vi "05TRM500_V2.vi"() -> ()   [LabVIEW 2020]
uses:
  <vilib>/Utility/error.llb/DialogType.ctl
  <vilib>/DAQmx/read.llb/DAQmx Read (Digital 1D U8 1Chan NSamp).vi
  <vilib>/Instr/_visa.llb/VISA Configure Serial Port (Serial Instr).vi
  <vilib>/DAQmx/create/channels.llb/DAQmx Create Channel (DI-Digital Input).vi
  <vilib>/DAQmx/configure/timing.llb/DAQmx Timing (Change Detection).vi
  <vilib>/DAQmx/miscellaneous.llb/DAQmx Fill In Error Info.vi
  <vilib>/ErrorRing/Error Ring.xnode
panel:
  in  "lines":tag="cDAQ1Mod1/port0/line0"
  in  "Tab Control":T1(tab)
  in  "INC DOWN":bool
  in  "INC UP":bool
  in  "MPH DOWN":bool
  in  "MPH UP":bool
  out "INC":dbl min=0.0 max=12.0 step=0.1 format="%.1g"
  out "MPH":dbl min=0.0 max=12.0 step=0.1 format="%.1g"
  out "Reply":string
  out "Error":string
  out "Directory":path
  out "Stopping":bool
  in  "Command":string
  in  "Insert Command":bool
  in  "Wait":bool
  out "Part":string
  in  "STOP":bool
  in  "Port":refnum<visa-resource-name>="COM8"
  in  "milliseconds to wait":u32
  out "Data":T2
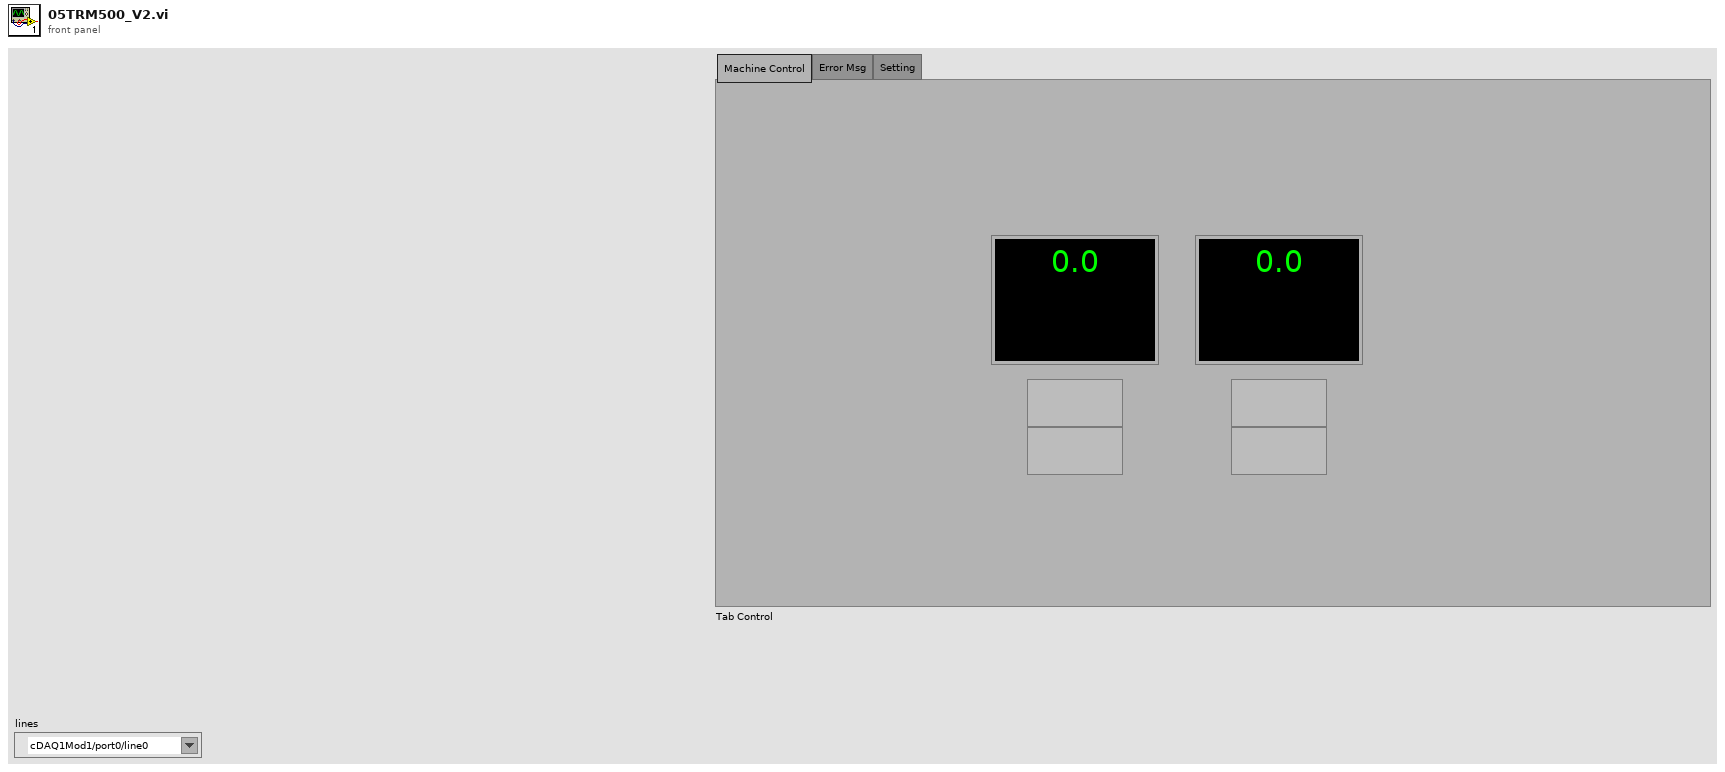
[diagram p1: front panel]
types:
  T1 = enum32{"Machine Control", "Error Msg", "Setting"}
  T2 = cluster{"err":i32[], "vin":i32, "vbus":i32, "amps":i32, "iamp":i32, "mph":i32, "inc":i32}
  T3 = enum16{"Initialize", "Next", "Send RSET", "Set MPH", "Set INC", "Part to 0"}
  T4 = enum16{"err", "mph:", "inc:", "cnfg:", "loop:", "type", "ver", "part:", "led2:", "xmph", "led1", "ptmp", "mtmp", "vbus", "iamp", "vin", "amps", "RSET", "ramp:", "res:", "rng:", "rpm"}[]
  T5 = typedef "DialogType.ctl" = u16
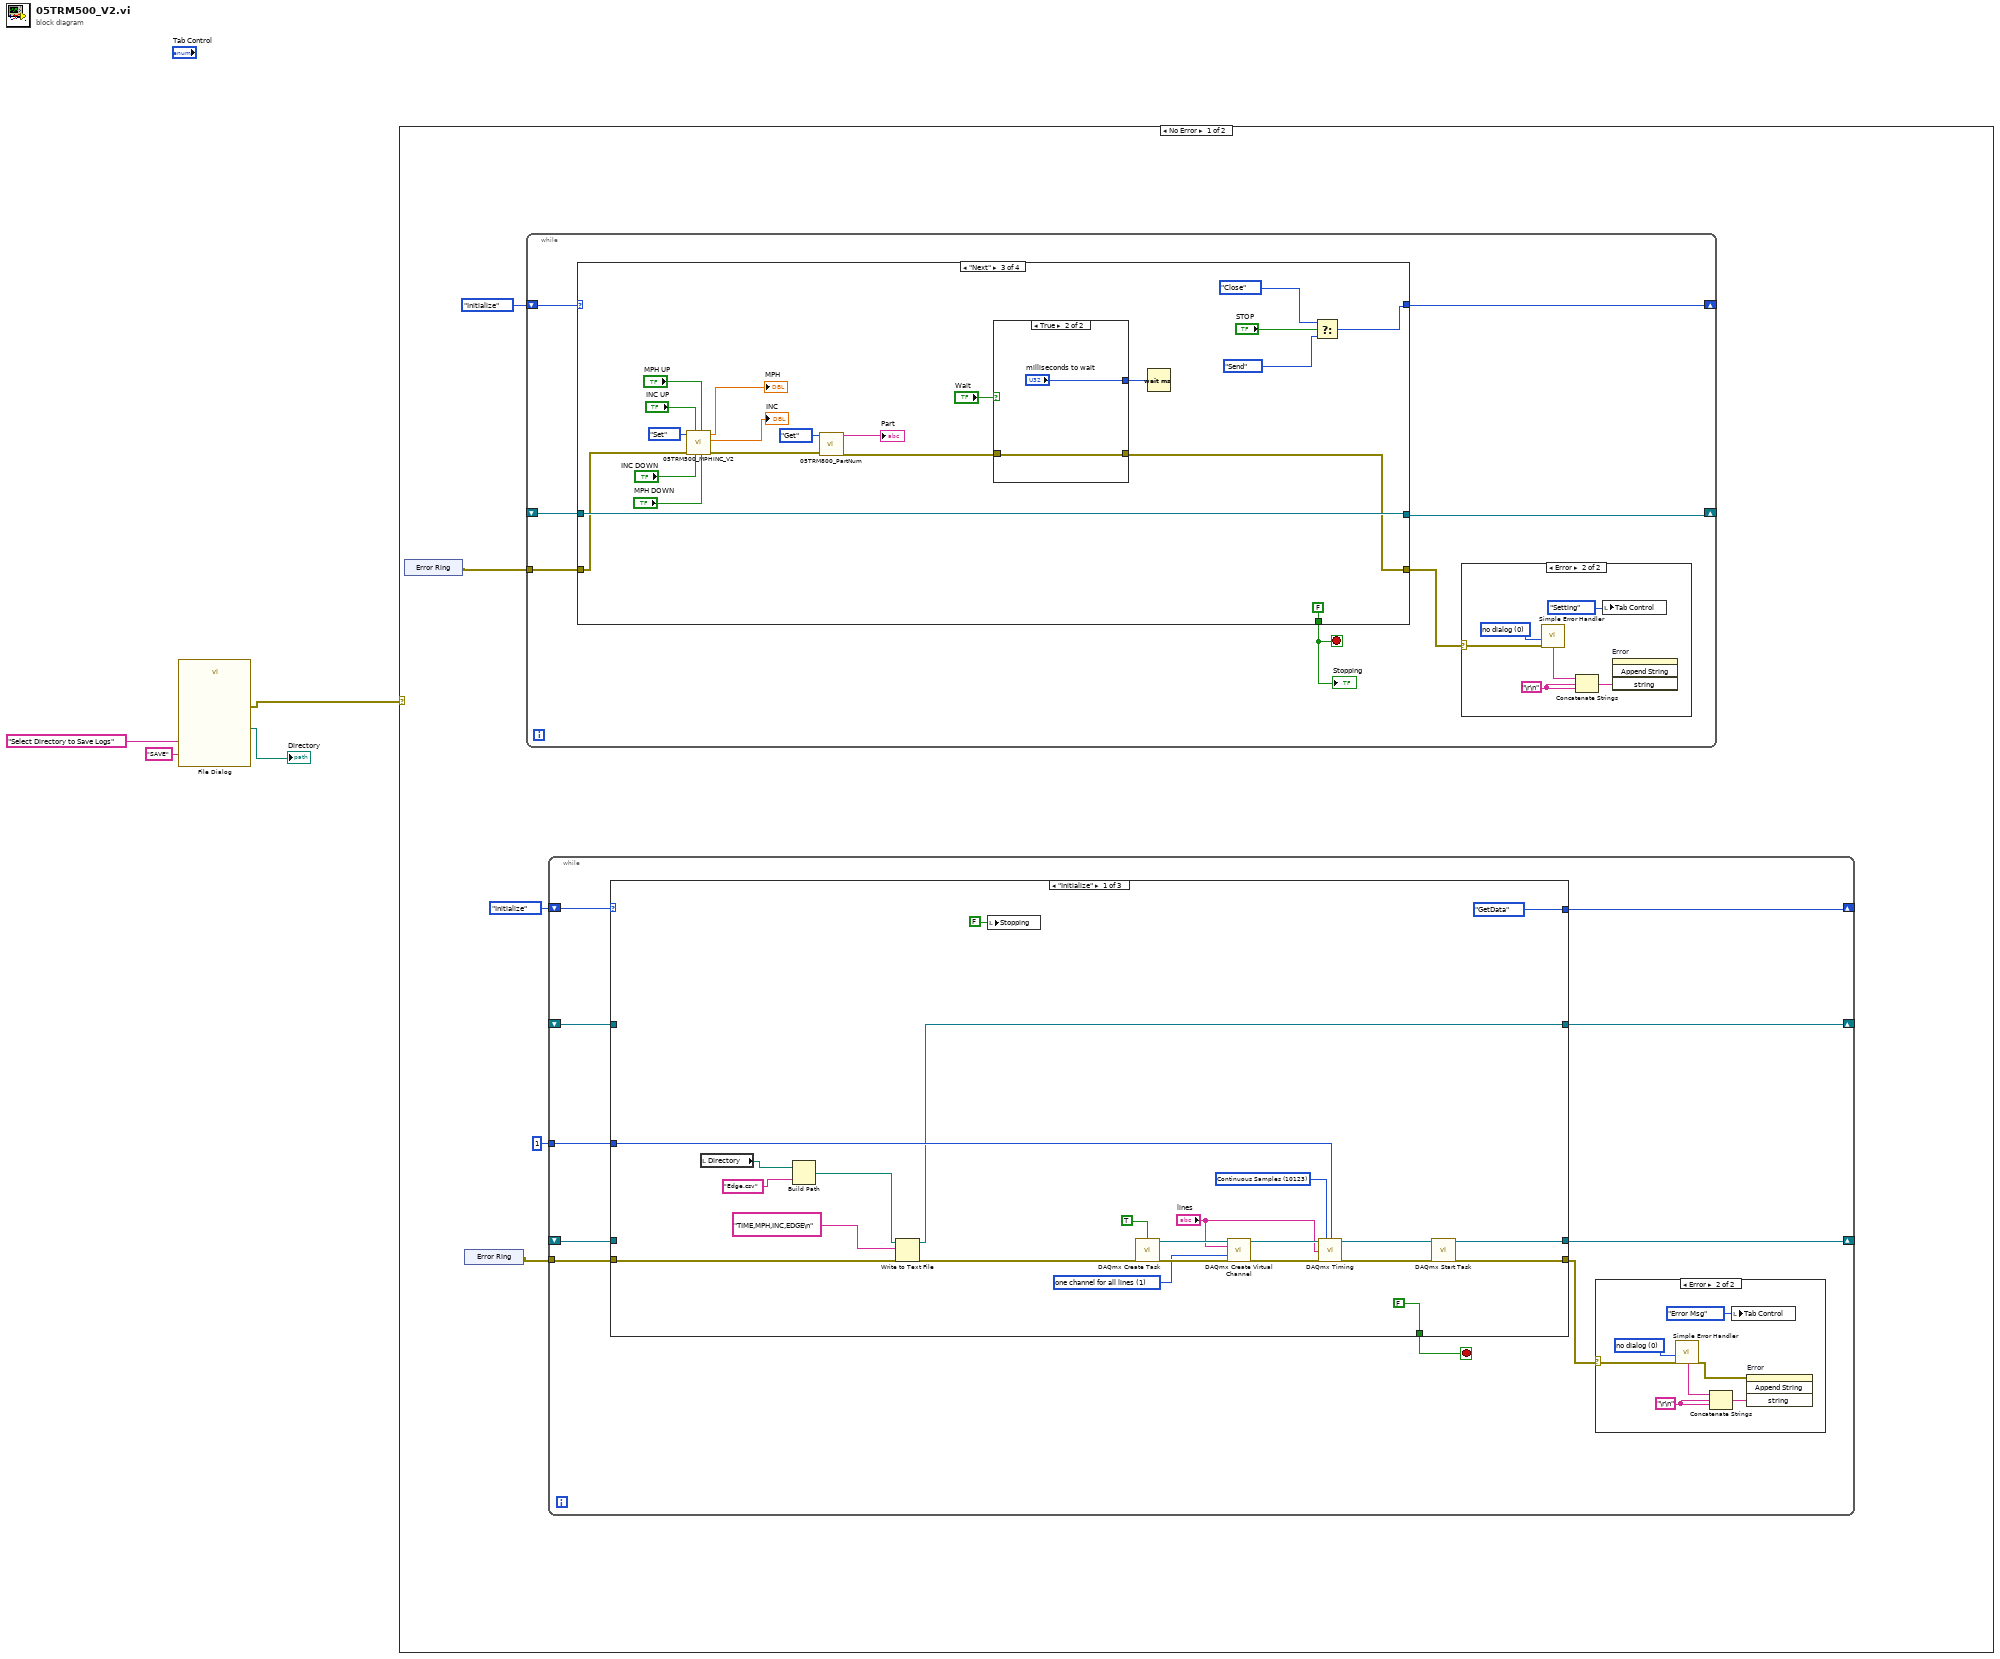
[diagram p0: block diagram]
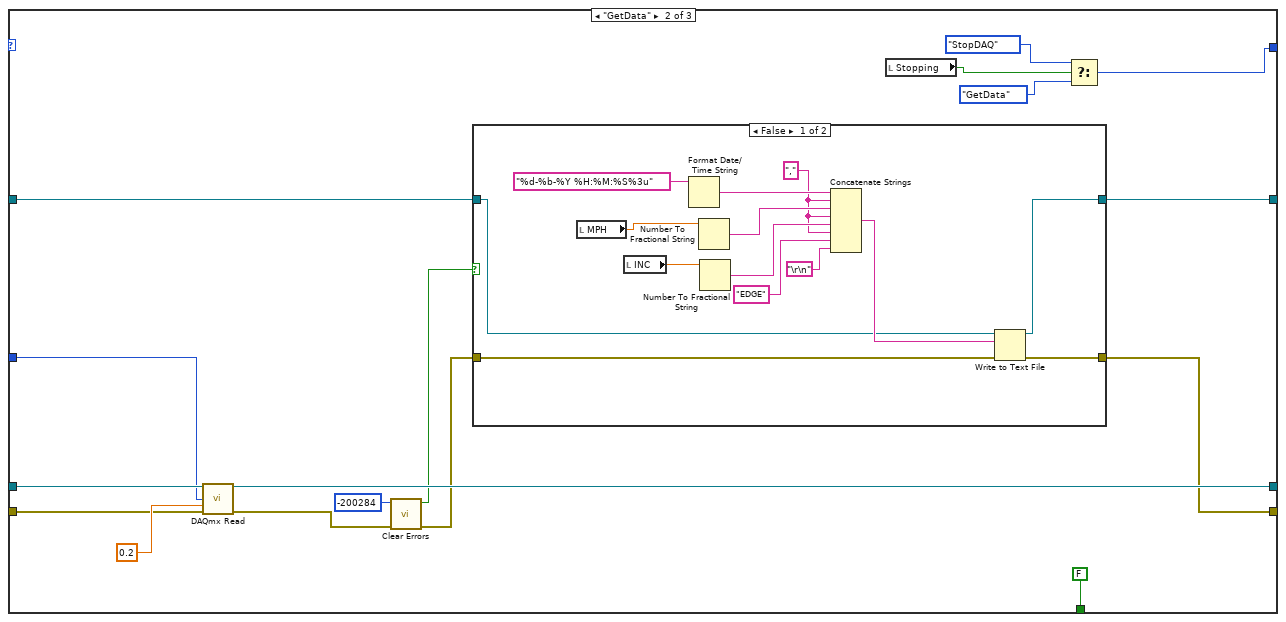
[diagram p3: hidden frame]
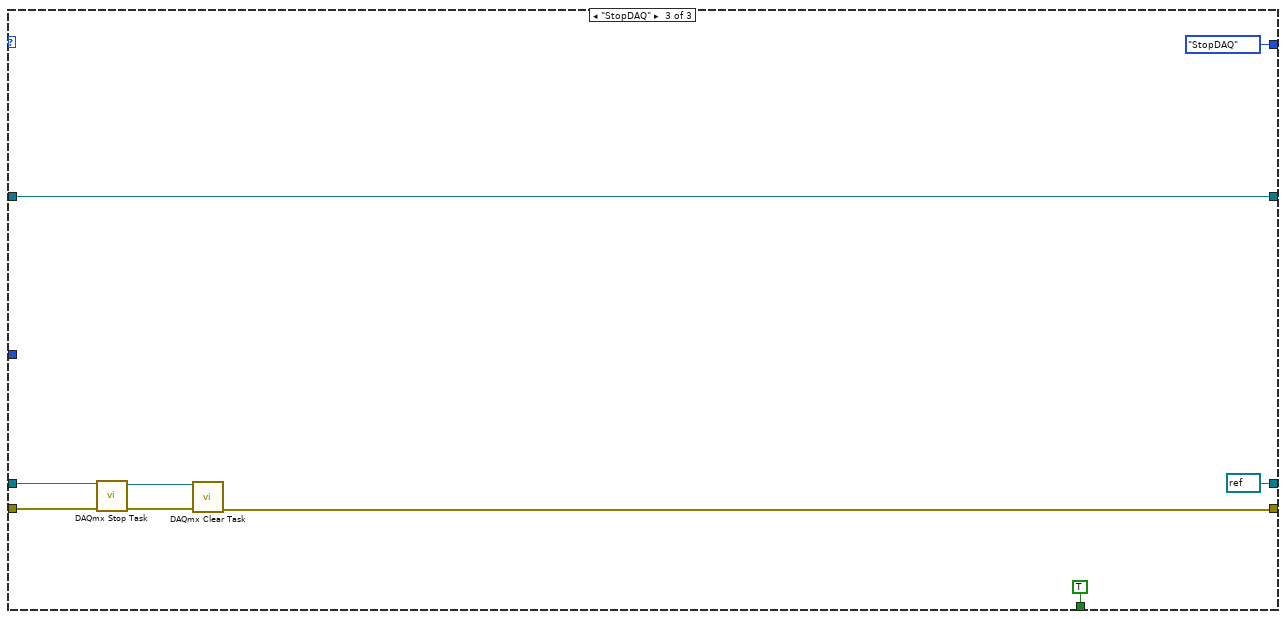
[diagram p5: hidden frame]
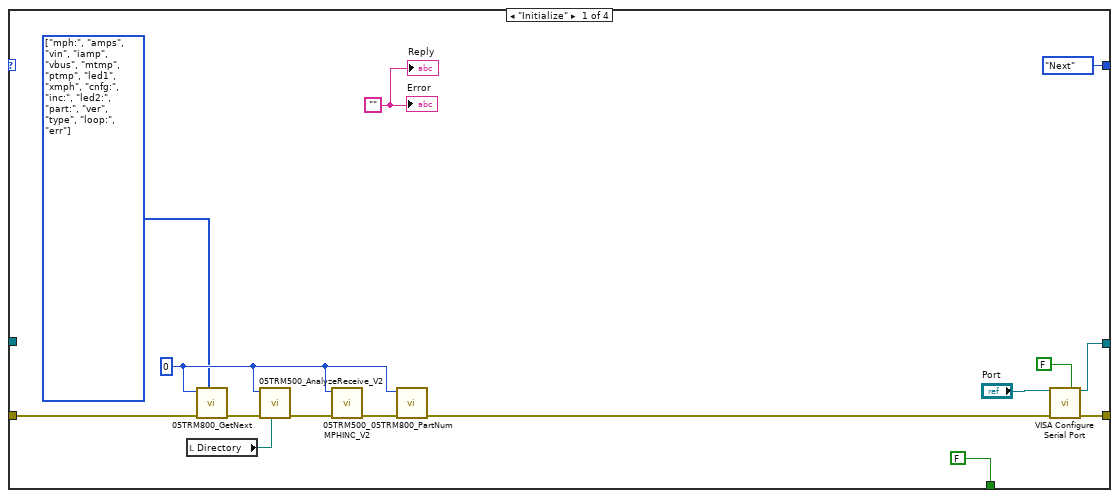
[diagram p7: hidden frame]
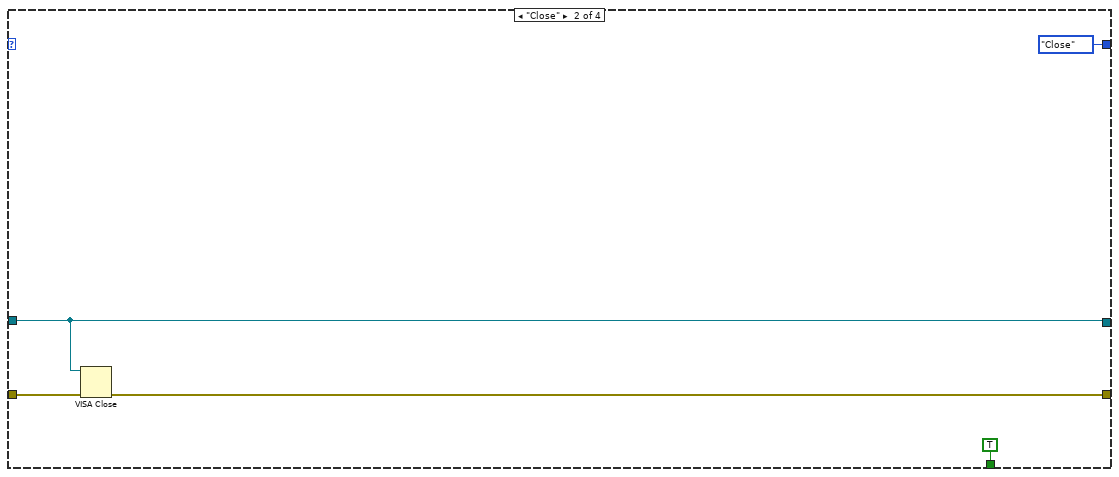
[diagram p8: hidden frame]
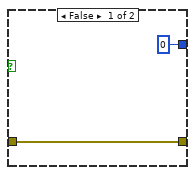
[diagram p9: hidden frame]
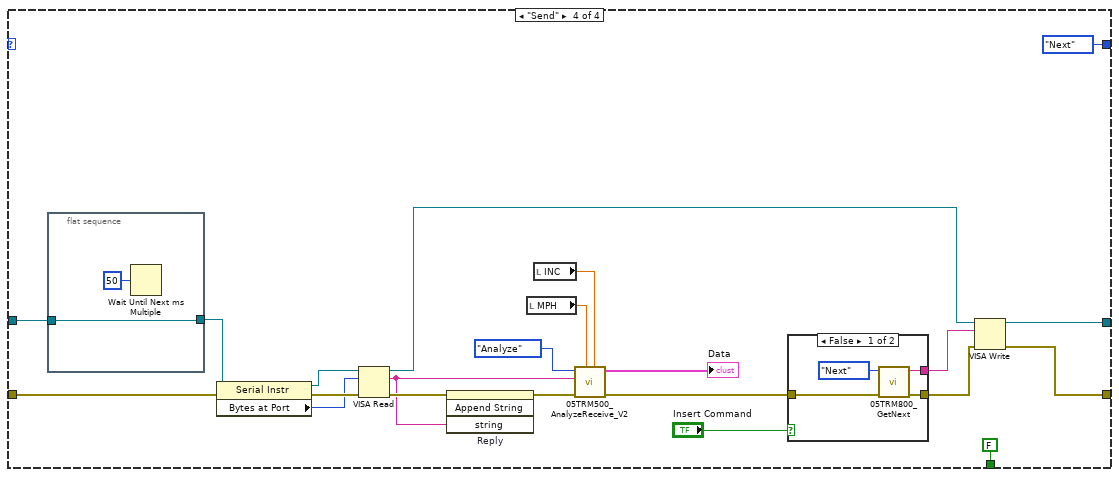
[diagram p10: hidden frame]
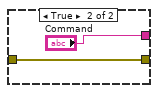
[diagram p11: hidden frame]
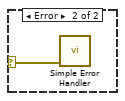
[diagram p12: hidden frame]
diagram:
  n1 = call "File Dialog"("prompt"="Select Directory to Save Logs", "button label"="SAVE") -> ("selected path"=→"Directory":path, "error out"=w4:errorcluster)  [unwired: 10 in, 2 out]
  n2 = case shown="No Error" w4 {
    selector: w4 -> [_ w182]
    frame No Error {
      n3 = xnode "Error Ring"() -> ("error out"=w6:errorcluster)
      n4 = xnode "Error Ring"() -> ("error out"=w5:errorcluster)
      n5 = while {
        shift-right: [w99] -> _
        shift-left: enum16{"Initialize", "Close", "Next", "Send"}."Initialize" -> [w100]
        tunnel: w6 -> [w98]
        shift-right: [w96] -> _
        shift-left: _ -> [w95]
        stop <- w94 stop-if-true
        n6 = case shown="\"Next\"" w100 {
          tunnel: [enum16{"Initialize", "Close", "Next", "Send"}."Next" enum16{"Initialize", "Close", "Next", "Send"}."Close" w145 enum16{"Initialize", "Close", "Next", "Send"}."Next"] -> w99
          tunnel: [FALSE TRUE FALSE FALSE] -> w94
          tunnel: w98 -> [w115 w125 w140 w171]
          tunnel: [w120 w123 w129 w164] -> w97
          tunnel: [w117 w124 w144 w165] -> w96
          tunnel: w95 -> [_ w124 w144 w173]
          frame "Initialize" {
            w109 = T4 [enum."mph:", enum."amps", enum."vin", enum."iamp", enum."vbus", enum."mtmp", enum."ptmp", enum."led1", enum."xmph", enum."cnfg:", enum."inc:", enum."led2:", enum."part:", enum."ver", enum."type", enum."loop:", enum."err"] items=["err", "mph:", "inc:", "cnfg:", "loop:", "type", "ver", "part:", "led2:", "xmph", "led1", "ptmp", "mtmp", "vbus", "iamp", "vin", "amps", "RSET", "ramp:", "res:", "rng:", "rpm"] ("Pattern")
            w112 = u16 0
            w116 = ""
            n7 = local read "Directory"() -> (w107:path)
            n8 = call "05TRM800_GetNext.vi"("Pattern"=w109, "error in (no error)"=w115, "Enum"=w112) -> ("error out"=w114:errorcluster)  [unwired: 7 in, 1 out]
            n9 = call "05TRM500_AnalyzeReceive_V2.vi"("Directory"=w107, "error in (no error)"=w114, "Enum"=w112) -> ("error out"=w113:errorcluster)  [unwired: 7 in, 1 out]
            n10 = call "05TRM500_MPHINC_V2.vi"("error in (no error)"=w113, "Enum"=w112) -> ("error out"=w111:errorcluster)  [unwired: 7 in, 2 out]
            n11 = call "05TRM800_PartNum.vi"("error in (no error)"=w111, "Enum"=w112) -> ("error out"=w110:errorcluster)  [unwired: 8 in, 1 out]
            n12 = call-poly "VISA Configure Serial Port"("VISA resource name"="Port", "Enable Termination\nChar (T)"=FALSE ("Enable Termination\nChar (T)"), "error in (no error)"=w110) -> ("VISA resource name out"=w117:refnum<visa-resource-name>, "error out"=w120:errorcluster)  [unwired: 11 in]
            "Error" <- w116
            "Reply" <- w116
          }
          frame "Close" {
            n13 = VISA Close(VISA resource name=w124, error in (no error)=w125) -> (error out=w123:errorcluster)
          }
          frame "Next" {
            n14 = call "05TRM500_MPHINC_V2.vi"("MPH DOWN"="MPH DOWN", "MPH UP"="MPH UP", "INC DOWN"="INC DOWN", "INC UP"="INC UP", "error in (no error)"=w140, "Enum"=enum16{"Initialize", "Set"}."Set") -> ("error out"=w133:errorcluster, "INC"=→"INC":dbl, "MPH"=→"MPH":dbl)  [unwired: 3 in]
            n15 = call "05TRM800_PartNum.vi"("error in (no error)"=w133, "Enum"=enum16{"Initialize", "Get", "Input"}."Get") -> ("error out"=w130:errorcluster, "Part Num"=→"Part":string)  [unwired: 8 in]
            n16 = case shown="True" "Wait" {
              tunnel: w130 -> [w149 w151]
              tunnel: [w149 w151] -> w129
              tunnel: [u32 0 ("milliseconds to wait") "milliseconds to wait"] -> w128
              frame False {
              }
              frame True {
              }
            }
            n17 = Wait (ms)(milliseconds to wait=w128) -> ()  [unwired: 1 out]
            n18 = Select(t=enum16{"Initialize", "Close", "Next", "Send"}."Close", s="STOP", f=enum16{"Initialize", "Close", "Next", "Send"}."Send") -> (s? t:f=w145:enum16{"Initialize", "Close", "Next", "Send"})
          }
          frame "Send" {
            n19 = flat-sequence {
              tunnel: w173 -> [w180]
              tunnel: [w180] -> w172
              frame #0 {
                n20 = Wait Until Next ms Multiple(millisecond multiple=u32 50) -> ()  [unwired: 1 out]
              }
            }
            n21 = property class="Serial Instr"(reference=w172, error in=w171) -> (reference out=w169:refnum<visa-resource-name>, error out=w170:errorcluster, "Bytes at Port"=w168:u32)
            n22 = VISA Read(VISA resource name=w169, byte count=w168, error in (no error)=w170) -> (VISA resource name out=w166:refnum<visa-resource-name>, read buffer=w157:string, error out=w167:errorcluster)  [unwired: 1 out]
            n23 = invoke on="Reply" class="Str" method="Append String"(error in=w167, "string"=w157) -> (error out=w159:errorcluster)  [unwired: 2 in, 3 out]
            n24 = local read "MPH"() -> (w153:dbl)
            n25 = local read "INC"() -> (w152:dbl)
            n26 = call "05TRM500_AnalyzeReceive_V2.vi"("INC"=w152, "MPH"=w153, "error in (no error)"=w159, "String"=w157, "Enum"=enum16{"Initialize", "Analyze"}."Analyze") -> ("error out"=w158:errorcluster, "Data"=→"Data":T2)  [unwired: 5 in]
            n27 = case shown="False" "Insert Command" {
              tunnel: [w177 "Command"] -> w161
              tunnel: [w176 w178] -> w160
              tunnel: w158 -> [w175 w178]
              frame False {
                n28 = call "05TRM800_GetNext.vi"("error in (no error)"=w175, "Enum"=T3."Next") -> ("error out"=w176:errorcluster, "String"=w177:string)  [unwired: 8 in]
              }
              frame True {
              }
            }
            n29 = VISA Write(VISA resource name=w166, write buffer=w161, error in (no error)=w160) -> (VISA resource name out=w165:refnum<visa-resource-name>, error out=w164:errorcluster)  [unwired: 1 out]
          }
        }
        "Stopping" <- w94
        n30 = case shown="Error" w97 {
          selector: w97 -> [_ w105]
          frame No Error {
          }
          frame Error {
            w102 = "\r\n"
            w106 = T5 0 items=["no dialog", "OK message", "continue or stop message", "OK message + warnings", "continue/stop + warnings"] ("type of dialog (OK msg:1)")
            n31 = call <vilib>:"Simple Error Handler.vi"("type of dialog (OK msg:1)"=w106, "error in (no error)"=w105) -> ("message"=w103:string)  [unwired: 3 in, 4 out]
            n32 = Concatenate Strings(w103, w102, w102) -> (w104:string)
            n33 = local write "Tab Control"(T1."Setting" ("Tab Control")) -> ()
            n34 = invoke on="Error" class="Str" method="Append String"("string"=w104) -> ()  [unwired: 3 in, 4 out]
          }
        }
      }
      n35 = while {
        shift-right: [w16] -> _
        shift-left: enum16{"Initialize", "GetData", "StopDAQ"}."Initialize" ("f") -> [w17]
        shift-right: [w20] -> _
        shift-left: _ -> [w19]
        tunnel: 1 ("samples per channel") -> [w18]
        tunnel: w5 -> [w14]
        shift-right: [w13] -> _
        shift-left: _ -> [w12]
        stop <- w21 stop-if-true
        n36 = case shown="\"Initialize\"" w17 {
          tunnel: [FALSE FALSE TRUE] -> w21
          tunnel: [w38 w61 refnum<k21> refnum ("task out")] -> w20
          tunnel: [w39 w54 w88] -> w15
          tunnel: w19 -> [_ w64 w91]
          tunnel: w14 -> [w32 w63 w92]
          tunnel: w18 -> [w44 w62 _]
          tunnel: [enum16{"Initialize", "GetData", "StopDAQ"}."GetData" ("f") w59 enum16{"Initialize", "GetData", "StopDAQ"}."StopDAQ" ("f")] -> w16
          tunnel: [w29 w53 w85] -> w13
          tunnel: w12 -> [_ w52 w85]
          frame "Initialize" {
            w43 = 10123 items=["Finite Samples"=10178, "Continuous Samples"=10123, "Hardware Timed Single Point"=12522] ("sample mode")
            w49 = 1 items=["one channel for each line", "one channel for all lines"] ("line grouping")
            n37 = local read "Directory"() -> (w30:path)
            n38 = Build Path(base path=w30, name or relative path="Edge.csv") -> (appended path=w33:path)
            n39 = Write to Text File(file (use dialog)=w33, text="TIME,MPH,INC,EDGE\n", error in=w32) -> (refnum out=w29:refnum<file>, error out=w31:errorcluster)  [unwired: 1 in, 1 out]
            n40 = local write "Stopping"(FALSE ("Stopping")) -> ()
            n41 = call <vilib>:"DAQmx Create Task.vi"("auto cleanup"=TRUE, "error in"=w31) -> ("task out"=w51:refnum<k21>, "error out"=w50:errorcluster)  [unwired: 12 in]
            n42 = call-poly <vilib>:"DAQmx Create Virtual Channel.vi"("task in"=w51, "lines"="lines", "line grouping"=w49, "error in"=w50) -> ("task out"=w45:refnum<k21>, "error out"=w46:errorcluster)  [unwired: 10 in]
            n43 = call-poly <vilib>:"DAQmx Timing.vi"("task/channels in"=w45, "sample mode"=w43, "samples per channel"=w44, "rising edge physical channels"="lines", "error in"=w46) -> ("task out"=w41:refnum<k21>, "error out"=w40:errorcluster)  [unwired: 9 in]
            n44 = call <vilib>:"DAQmx Start Task.vi"("task/channels in"=w41, "error in"=w40) -> ("task out"=w38:refnum<k21>, "error out"=w39:errorcluster)  [unwired: 12 in]
          }
          frame "GetData" {
            n45 = call-poly <vilib>:"DAQmx Read.vi"("task/channels in"=w64, "number of samples per channel"=w62, "timeout"=0.2, "error in"=w63) -> ("task out"=w61:refnum<k21>, "error out"=w65:errorcluster)  [unwired: 9 in, 1 out]
            n46 = call <vilib>:"Clear Errors.vi"("error in (no error)"=w65, "specific error code to clear (0: all)"=-200284) -> ("error out"=w55:errorcluster, "specific error cleared?"=w56:bool)  [unwired: 4 in]
            n47 = case shown="False" w56 {
              tunnel: w55 -> [w75 w84]
              tunnel: [w74 w84] -> w54
              tunnel: [w69 w83] -> w53
              tunnel: w52 -> [w70 w83]
              frame False {
                w76 = ","
                n48 = local read "MPH"() -> (w72:dbl)
                n49 = local read "INC"() -> (w73:dbl)
                n50 = Format Date/Time String(time format string (%c)="%d-%b-%Y %H:%M:%S%3u") -> (date/time string=w81:string)  [unwired: 2 in]
                n51 = Number To Fractional String(number=w72) -> (F-format string=w80:string)  [unwired: 3 in]
                n52 = Number To Fractional String(number=w73) -> (F-format string=w79:string)  [unwired: 3 in]
                n53 = Concatenate Strings(w81, w76, w80, w76, w79, w76, "EDGE", "\r\n") -> (w78:string)
                n54 = Write to Text File(file (use dialog)=w70, text=w78, error in=w75) -> (refnum out=w69:refnum<file>, error out=w74:errorcluster)  [unwired: 1 in, 1 out]
              }
              frame True {
              }
            }
            n55 = local read "Stopping"() -> (w57:bool)
            n56 = Select(t=enum16{"Initialize", "GetData", "StopDAQ"}."StopDAQ", s=w57, f=enum16{"Initialize", "GetData", "StopDAQ"}."GetData") -> (s? t:f=w59:enum16{"Initialize", "GetData", "StopDAQ"})
          }
          frame "StopDAQ" {
            n57 = call <vilib>:"DAQmx Stop Task.vi"("task/channels in"=w91, "error in"=w92) -> ("task out"=w89:refnum<k21>, "error out"=w90:errorcluster)  [unwired: 12 in]
            n58 = call <vilib>:"DAQmx Clear Task.vi"("task in"=w89, "error in"=w90) -> ("error out"=w88:errorcluster)  [unwired: 13 in]
          }
        }
        n59 = case shown="Error" w15 {
          selector: w15 -> [_ w27]
          frame No Error {
          }
          frame Error {
            w24 = "\r\n"
            w28 = T5 0 items=["no dialog", "OK message", "continue or stop message", "OK message + warnings", "continue/stop + warnings"] ("type of dialog (OK msg:1)")
            n60 = call <vilib>:"Simple Error Handler.vi"("type of dialog (OK msg:1)"=w28, "error in (no error)"=w27) -> ("error out"=w23:errorcluster, "message"=w25:string)  [unwired: 3 in, 3 out]
            n61 = Concatenate Strings(w25, w24, w24) -> (w26:string)
            n62 = local write "Tab Control"(T1."Error Msg" ("Tab Control")) -> ()
            n63 = invoke on="Error" class="Str" method="Append String"(error in=w23, "string"=w26) -> ()  [unwired: 2 in, 4 out]
          }
        }
      }
    }
    frame Error {
      n64 = call <vilib>:"Simple Error Handler.vi"("error in (no error)"=w182) -> ()  [unwired: 4 in, 5 out]
    }
  }
